vi "Extract Multiple Tone Information 1 Chan.vi"(0 "time signal in":waveform(dbl), 5 "export mode":T3(ring), 7 "threshold":dbl=0.001 format="%#_6p", 9 "max num tones":i32=4, 11 "error in (no error)":errorcluster, 12 "output sorting":i32(ring) items=["increasing frequency", "decreasing amplitude"]) -> (3 "exported signals":T2 {"exported spectrum (dB)"."dB Spectrum (Hann)" format="%.2p"; "exported spectrum (dB)"."df" format="%.2p"; "exported spectrum (dB)"."f0" format="%.2p"}, 4 "multiple tone information":T1(array[cluster]) {"detected phase (deg)" format="%_6g"; "detected amplitude" format="%_6p"; "detected frequency" format="%_6p"}, 15 "error out":errorcluster)   [LabVIEW 2020, in "NI_MAPro.lvlib"]
doc: "Returns the frequency, amplitude, and phase for each signal tone whose amplitude exceeds a specified <B>threshold</B>. Wire data to the <B>time signal in</B> input to determine the polymorphic instance to use or manually select the instance."
uses:
  NI_MAPro.lvlib
  ma_sml_Spectrum Cluster (complex).ctl
  ma_sml_Spectral Info.ctl
  NI_MABase.lvlib
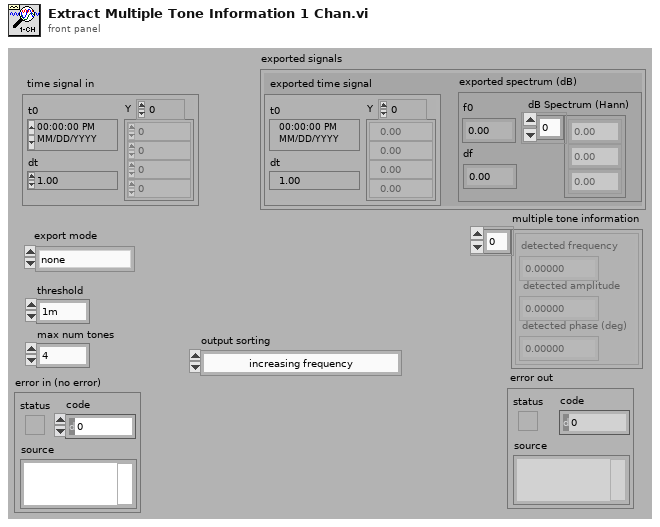
[diagram p1: front panel]
types:
  T1 = cluster{"detected frequency":dbl, "detected amplitude":dbl, "detected phase (deg)":dbl}[]
  T2 = cluster{"exported time signal":waveform(dbl), "exported spectrum (dB)":cluster{"f0":dbl, "df":dbl, "dB Spectrum (Hann)":dbl[]}}
  T3 = enum32{"none", "input signal", "detected signal", "residual signal"}
  T4 = typedef "NI_MAPro.lvlib/ma_sml_Spectrum Cluster (complex).ctl" = cluster{"f0":dbl, "df":dbl, "spectrum":cdb[]}
  T5 = typedef "NI_MAPro.lvlib/ma_sml_Spectral Info.ctl" = cluster{"spectrum type":enum16{"FFT Spectrum [complex]", "Amplitude [Magnitude]", "Power [Magnitude^2]", "Cross Spectrum [complex]", "Frequency Response [Complex]"}, "linear/dB":enum16{"linear", "dB"}, "window":u16, "window size":i32, "FFT size":i32}
  T6 = cluster{"frequency [Hz]":dbl, "magnitude":dbl, "phase [degree]":dbl}
  T7 = cluster{"Single/Multiple":enum16{"Multiple Peaks", "Single Max Peak"}, "Threshold":dbl, "max #tones":i32}
  T8 = cluster{"f0":dbl, "df":dbl, "dB Spectrum (Hann)":dbl[]}
  T9 = cluster{"frequency [Hz]":dbl, "amplitude":dbl, "phase [degree]":dbl}[]
  T10 = cluster{waveform(dbl), "exported spectrum (dB)":cluster{"f0":dbl, "df":dbl, "dB Spectrum (Hann)":dbl[]}}
  T11 = cluster{"time signal in":waveform(dbl), cluster{dbl, dbl, dbl[]}}
  T12 = cluster{"time signal in":waveform(dbl), cluster{dbl, dbl, "Y":dbl[]}}
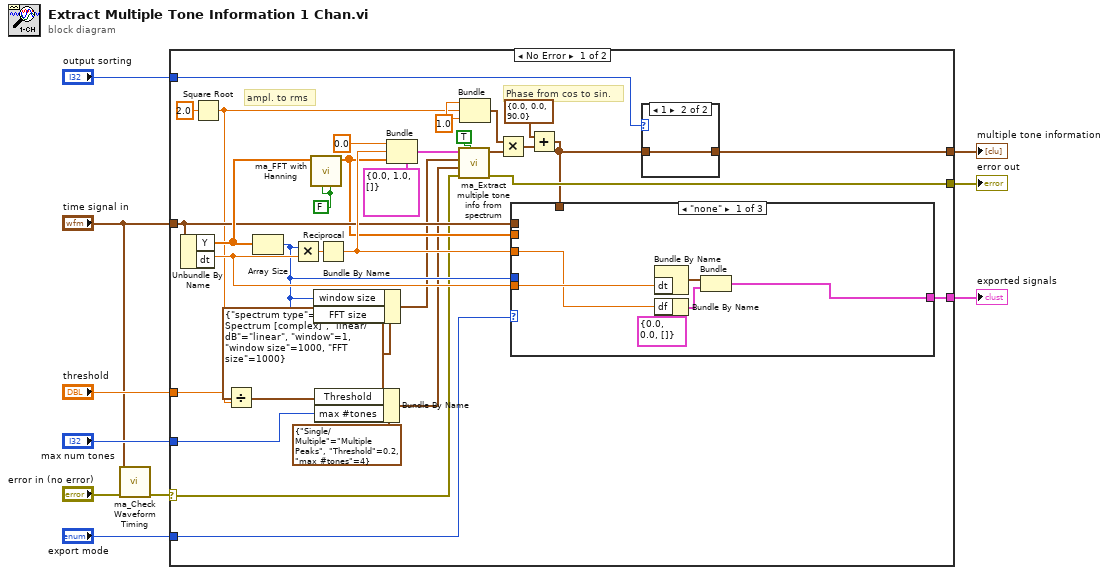
[diagram p0: block diagram]
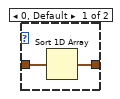
[diagram p2: hidden frame]
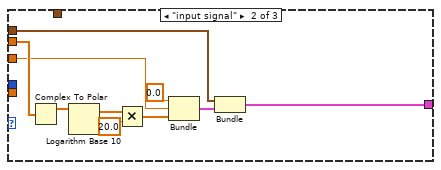
[diagram p3: hidden frame]
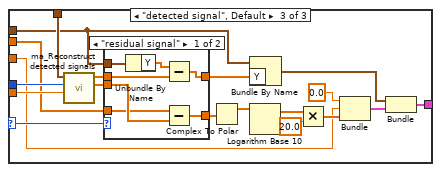
[diagram p4: hidden frame]
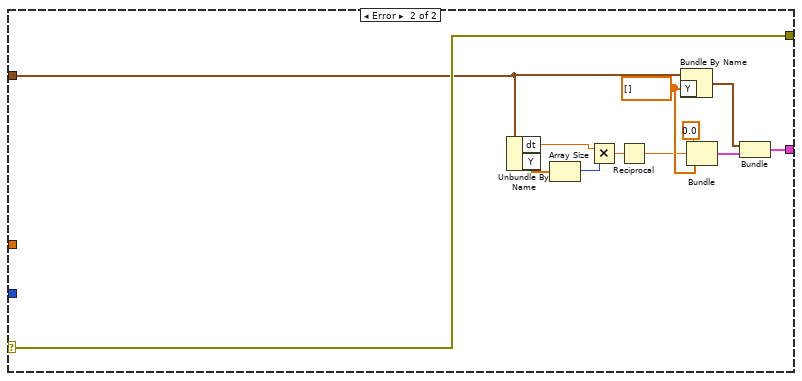
[diagram p6: hidden frame]
diagram:
  n1 = call "ma_Check Waveform Timing.vi"("error in (no error)"="error in (no error)", "signal in"="time signal in") -> ("error out"=w1:errorcluster)  [unwired: 1 in, 8 out]
  n2 = case shown="No Error" w1 {
    selector: w1 -> [w27 w102]
    tunnel: "export mode" -> [w15 _]
    tunnel: [w39 w101] -> w9
    tunnel: "time signal in" -> [w36 w99]
    tunnel: [w33 w102] -> w8
    tunnel: "max num tones" -> [w30 _]
    tunnel: "threshold" -> [w25 _]
    tunnel: "output sorting" -> [w29 _]
    tunnel: [w28 _] -> w4
    frame No Error {
      w18 = 1.0
      w16 = FALSE ("correct DC")
      # "Phase from cos to sin."
      # "ampl. to rms"
      n3 = Unbundle By Name(w36) -> ("Y"=w41:dbl[], "dt"=w38:dbl)
      n4 = Square Root(x=2.0) -> (sqrt(x)=w17:dbl)
      n5 = Divide(x=w25, y=w17) -> (x/y=w24:dbl)
      n6 = Array Size(array=w41) -> (size(s)=w34:i32)
      n7 = Multiply(x=w34, y=w38) -> (x*y=w43:dbl)
      n8 = call "ma_FFT with Hanning.vi"("exclude Nyquist"=w16, "correct DC"=w16, "time signal data"=w41) -> ("complex Hann spectrum"=w35:cdb[])  [unwired: 2 in, 6 out]
      n9 = Bundle By Name(cluster=T5 {"spectrum type"=enum."FFT Spectrum [complex]", "linear/dB"=enum."linear", "window"=1, "window size"=1000, "FFT size"=1000} ("spectral info"), "window size"=w34, "FFT size"=w34) -> (w11:T5)
      n10 = Bundle By Name(cluster=T7 {"Single/Multiple"=enum."Multiple Peaks", "Threshold"=0.2, "max #tones"=4} ("criterion"), "Threshold"=w24, "max #tones"=w30) -> (w32:T7)
      n11 = Reciprocal(x=w43) -> (1/x=w37:dbl)
      n12 = Bundle(cluster=T4 {"f0"=0.0, "df"=1.0, "spectrum"=[]} ("FFT spectrum"), "f0"=0.0, "df"=w37, "spectrum"=w35) -> (w13:T4)
      n13 = call "ma_Extract multiple tone info from spectrum.vi"("spectrum includes end points?"=TRUE, "error in"=w27, "criterion"=w32, "spectral info"=w11, "FFT spectrum"=w13) -> ("error out"=w33:errorcluster, "extracted tones (sorted by amplitude)"=w23:T9)  [unwired: 1 in, 4 out]
      n14 = Bundle(w18, w17, w18) -> (w19:cluster{dbl, dbl, dbl})  [unwired: 1 out]
      n15 = Multiply(x=w19, y=w23) -> (x*y=w22:cluster{dbl, dbl, dbl}[])
      n16 = Add(x=T6 {"frequency [Hz]"=0.0, "magnitude"=0.0, "phase [degree]"=90.0} ("single tone info."), y=w22) -> (x+y=w21:cluster{dbl, dbl, dbl}[])
      n17 = case shown="\"none\"" w15 {
        selector: w15 -> [_ _ w78]
        tunnel: w21 -> [_ _ w81]
        tunnel: [w49 w62 w63] -> w39
        tunnel: w38 -> [w48 _ w80]
        tunnel: w37 -> [w47 w53 w64]
        tunnel: w36 -> [_ w61 w66]
        tunnel: w35 -> [_ w54 w75]
        tunnel: w34 -> [_ _ w79]
        frame "none" {
          n18 = Bundle By Name("dt"=w48) -> (w52:waveform(dbl))  [unwired: 1 out]
          n19 = Bundle By Name(cluster=T8 {"f0"=0.0, "df"=0.0, "dB Spectrum (Hann)"=[]} ("exported spectrum (dB)"), "df"=w47) -> (w50:T8)
          n20 = Bundle(w52, "exported spectrum (dB)"=w50) -> (w49:T10)  [unwired: 1 out]
        }
        frame "input signal" {
          n21 = Complex To Polar(r * e^(i*theta)=w54) -> (r=w60:dbl[])  [unwired: 1 out]
          n22 = Logarithm Base 10(1:w60) -> (0:w59:dbl[])
          n23 = Multiply(x=w59, y=20.0) -> (x*y=w55:dbl[])
          n24 = Bundle(0.0, w53, w55) -> (w56:cluster{dbl, dbl, dbl[]})  [unwired: 1 out]
          n25 = Bundle("time signal in"=w61, w56) -> (w62:T11)  [unwired: 1 out]
        }
        frame "detected signal", Default {
          n26 = call "ma_Reconstruct detected signals.vi"("dt"=w80, "# samples"=w79, "multiple tone information"=w81) -> ("detected Hann spectrum"=w76:cdb[], "detected time array"=w77:dbl[])  [unwired: 7 out]
          n27 = case shown="\"residual signal\"" w78 {
            tunnel: w77 -> [w88 w89]
            tunnel: [w83 w90] -> w68
            tunnel: w76 -> [w84 w90]
            tunnel: w66 -> [w87 _]
            tunnel: [w85 w89] -> w67
            tunnel: w75 -> [w82 _]
            frame "residual signal" {
              n28 = Unbundle By Name(w87) -> ("Y"=w86:dbl[])
              n29 = Subtract(x=w86, y=w88) -> (x-y=w85:dbl[])
              n30 = Subtract(x=w82, y=w84) -> (x-y=w83:cdb[])
            }
            frame "detected signal", Default {
            }
          }
          n31 = Complex To Polar(r * e^(i*theta)=w68) -> (r=w74:dbl[])  [unwired: 1 out]
          n32 = Bundle By Name(cluster=w66, "Y"=w67) -> (w65:waveform(dbl))
          n33 = Logarithm Base 10(1:w74) -> (0:w73:dbl[])
          n34 = Multiply(x=w73, y=20.0) -> (x*y=w69:dbl[])
          n35 = Bundle(0.0, w64, w69) -> (w70:cluster{dbl, dbl, dbl[]})  [unwired: 1 out]
          n36 = Bundle("time signal in"=w65, w70) -> (w63:T11)  [unwired: 1 out]
        }
      }
      n37 = case shown="1" w29 {
        tunnel: [w44 w46] -> w28
        tunnel: w21 -> [w45 w46]
        frame 0, Default {
          n38 = Sort 1D Array(array=w45) -> (sorted array=w44:cluster{dbl, dbl, dbl}[])
        }
        frame 1 {
        }
      }
    }
    frame Error {
      w96 = dbl[] [] ("Y")
      n39 = Unbundle By Name(w99) -> ("dt"=w93:dbl, "Y"=w95:dbl[])
      n40 = Array Size(array=w95) -> (size(s)=w94:i32)
      n41 = Multiply(x=w93, y=w94) -> (x*y=w92:dbl)
      n42 = Reciprocal(x=w92) -> (1/x=w91:dbl)
      n43 = Bundle By Name(cluster=w99, "Y"=w96) -> (w100:waveform(dbl))
      n44 = Bundle(0.0, w91, "Y"=w96) -> (w98:cluster{dbl, dbl, "Y":dbl[]})  [unwired: 1 out]
      n45 = Bundle("time signal in"=w100, w98) -> (w101:T12)  [unwired: 1 out]
    }
  }
  "error out" <- w8
  "exported signals" <- w9
  "multiple tone information" <- w4
